vi "DHE_get_shutter_pos.vi"(0 "fd":i32, 11 "error in (no error)":errorcluster) -> (4 "fd out":i32, 8 "shutter":i32, 15 "error out":errorcluster)   [LabVIEW 2016]
doc: "This VI turns instrument power on (Flag=1) or off (Flag=0)."
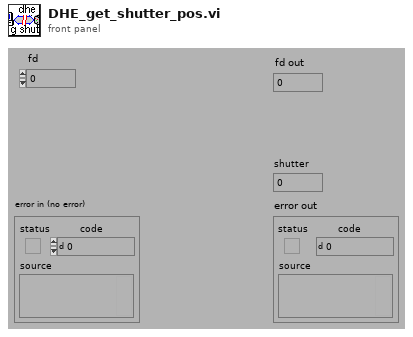
[diagram p1: front panel]
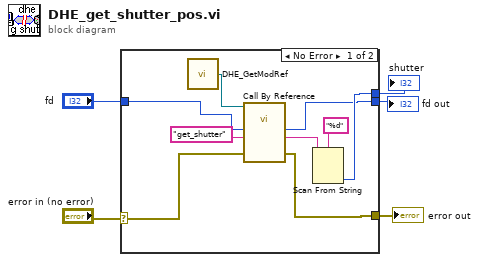
[diagram p0: block diagram]
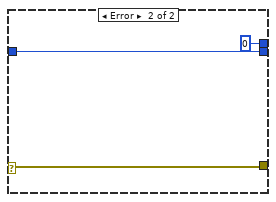
[diagram p2: hidden frame]
diagram:
  n1 = case shown="No Error" "error in (no error)" {
    selector: "error in (no error)" -> [w9 w15]
    tunnel: "fd" -> [w10 w17]
    tunnel: [w7 0] -> w4
    tunnel: [w8 w15] -> w3
    tunnel: [w6 w17] -> w2
    frame No Error {
      n2 = call "DHE_GetModRef.vi"() -> ("DHE_ModRef"=w14:refnum<vi>)  [unwired: 9 out]
      n3 = call-by-ref "?"(reference=w14, "error in (no error)"=w9, "function"="get_shutter", "fd in"=w10) -> ("error out"=w8:errorcluster, "str result"=w12:string, "fd out"=w6:i32)  [unwired: 6 in, 3 out]
      n4 = Scan From String(format string="%d", input string=w12) -> (output 1=w7:i32)  [unwired: 2 in, 4 out]
    }
    frame Error {
    }
  }
  "error out" <- w3
  "shutter" <- w4
  "fd out" <- w2
